vi "PrefDialog.vi"(8 "error in (no error)":errorcluster, 11 "MyPluginsBase in":refnum<class "AcPwrBase.lvclass">) -> (0 "error out":errorcluster, 1 "Save As":bool, 2 "Changed":bool, 3 "MyPluginsBase out":refnum<class "AcPwrBase.lvclass">)   [LabVIEW 2018, in "AcPwrPlugins.lvlib" / "AcPwrBase.lvclass"]
uses:
  AcPwrBase.lvclass
  C:/Program Files (x86)/National Instruments/LabVIEW 2018/user.lib/NIST/BaseClasses/BasePlugin_class/BasePlugin.lvclass
  TypeDefs/BaseConfig.ctl
  TypeDefs/Phase.ctl
  TypeDefs/BaseMeasurements.ctl
  TypeDefs/MeasType.ctl
  <userlib>/NIST/BaseClasses/BasePlugin_class/BasePlugin.lvclass/BasePlugin.ctl
  AcPwrBase.lvclass/AcPwrBase.ctl
  FGen/MemberClasses/FunctionBaseClass/FunctionBase.lvclass
  <userlib>/NIST/BaseClasses/BasePlugin_class/Accessors/Read PluginIniFilePath.vi
  Accessors/Read BaseConfig.vi
  Accessors/Read FunctionINIFilePath.vi
  Accessors/Read RefreshTime.vi
  Accessors/Read BaseMeasurements.vi
  Accessors/Read FunctionClass.vi
  Accessors/Write FunctionClass.vi
  Accessors/Write FunctionINIFilePath.vi
  Accessors/Write BaseConfig.vi
  Accessors/Write RefreshTime.vi
  Accessors/Write BaseMeasurements.vi
  <userlib>/NIST/BaseClasses/BasePlugin_class/Accessors/Write PluginIniFilePath.vi
  <vilib>/Utility/error.llb/Error Cluster From Error Code.vi
  <vilib>/ErrorRing/Error Ring.xnode
  <vilib>/Utility/config.llb/NI_LVConfig.lvlib
  <userlib>/NIST/BaseClasses/Object_class/BaseObject.lvclass
panel:
  in  "BaseMeasurements":T1
  in  "btnSaveAs":bool
  in  "btnSave":bool
  in  "RefreshTime":dbl
  in  "FunctionIniFilePath":path
  in  "btnFuncConfig":bool
  in  "btnCancel":bool
  in  "BaseConfig":T3
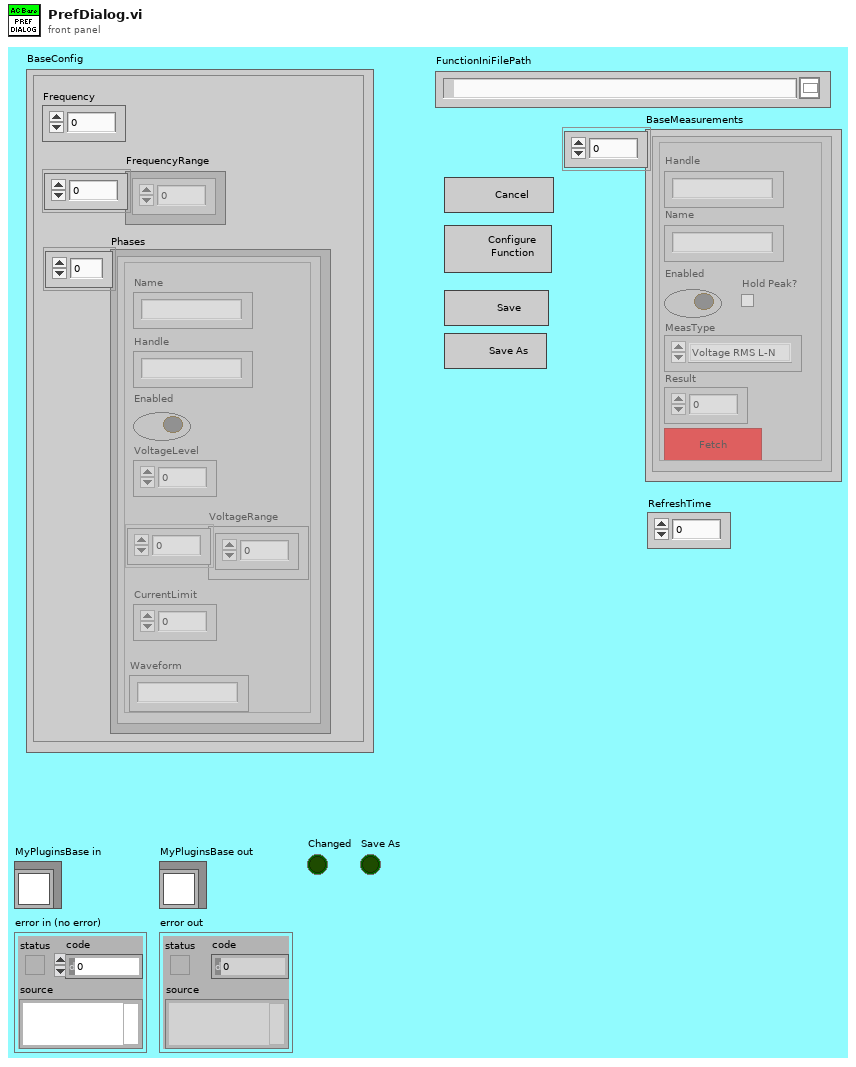
[diagram p1: front panel]
types:
  T1 = typedef "AcPwrPlugins.lvlib/AcPwrBase.lvclass/BaseMeasurements.ctl" = cluster{"Handle":string, "Name":string, "Enabled":bool, "Result":dbl, "MeasType":T2, "btnMeasFetch":bool, "Hold Peak?":bool}[]
  T2 = typedef "AcPwrPlugins.lvlib/AcPwrBase.lvclass/MeasType.ctl" = enum16{"Voltage RMS L-N", "Current RMS", "Frequency", "Voltage DC", "Current DC", "Power Factor", "Current Peak", "Power VA", "Real Power", "Voltage THD", "Voltage EHD", "Voltage OHD", "Current THD", "Current EHD", "Current OHD", "Voltage RMS L-L", "Phase Angle", "Power DC", "Crest Factor"}
  T3 = typedef "AcPwrPlugins.lvlib/AcPwrBase.lvclass/BaseConfig.ctl" = cluster{"Frequency":dbl, "FrequencyRange":dbl[], "Phases":T4[]}
  T4 = typedef "AcPwrPlugins.lvlib/AcPwrBase.lvclass/Phase.ctl" = cluster{"Name":string, "Enabled":bool, "VoltageLevel":dbl, "Handle":string, "VoltageRange":dbl[], "Connected":bool, "CurrentLimit":dbl, "Waveform":string}
  T5 = enum8{"Enabled", "Disabled", "Disabled and Grayed Out"}
  T6 = enum32{"Invalid", "Standard", "Closed", "Hidden", "Minimized", "Maximized"}
  T7 = enum32{"Invalid", "Default", "Floating", "Floating/Auto-Hide", "Modal"}
  T8 = typedef "NI_LVConfig.lvlib/Config Data RefNum.ctl" = refnum<k1>
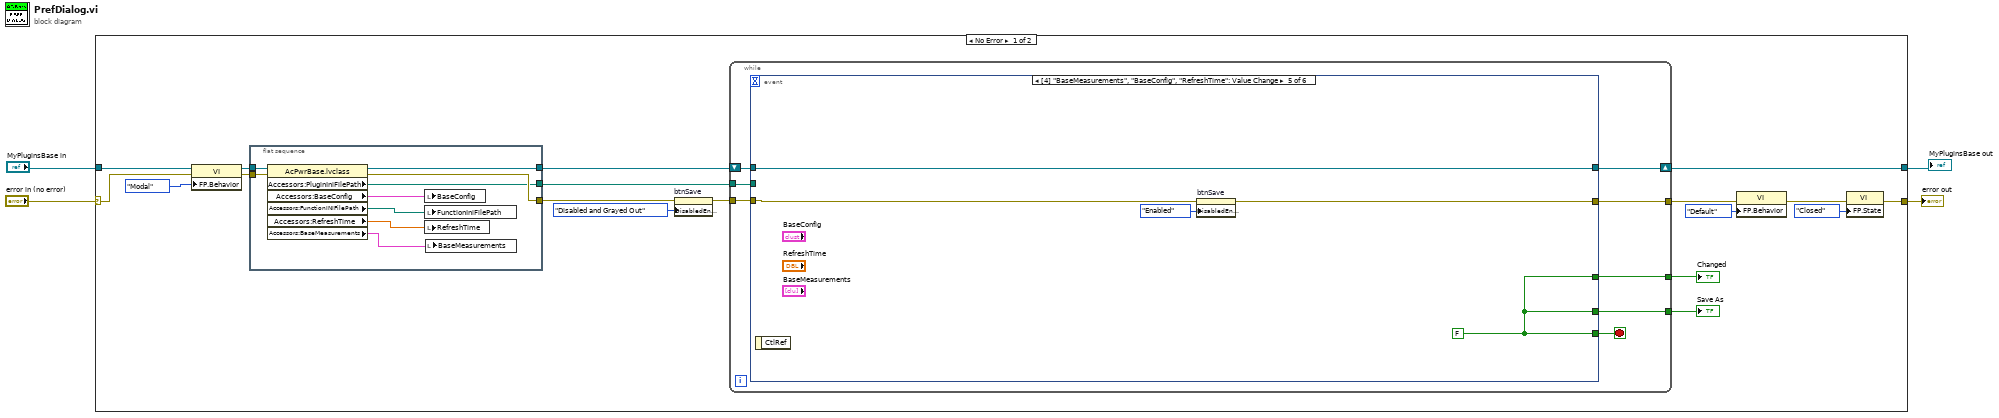
[diagram p0: block diagram]
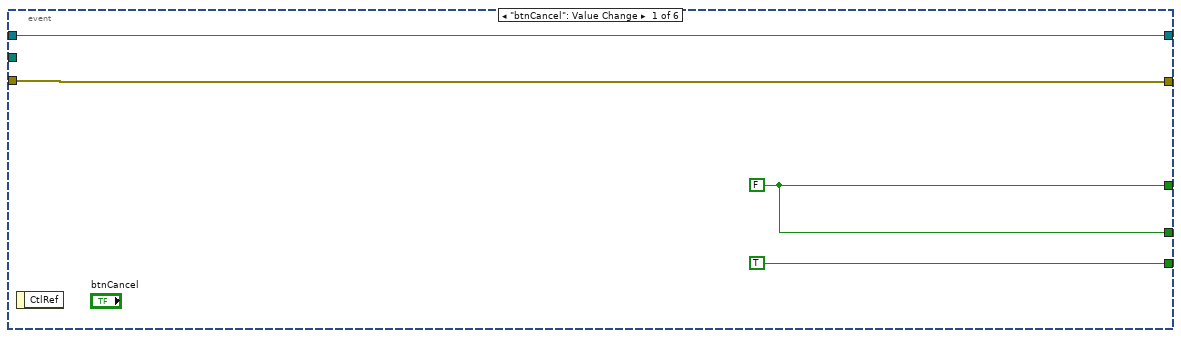
[diagram p2: hidden frame]
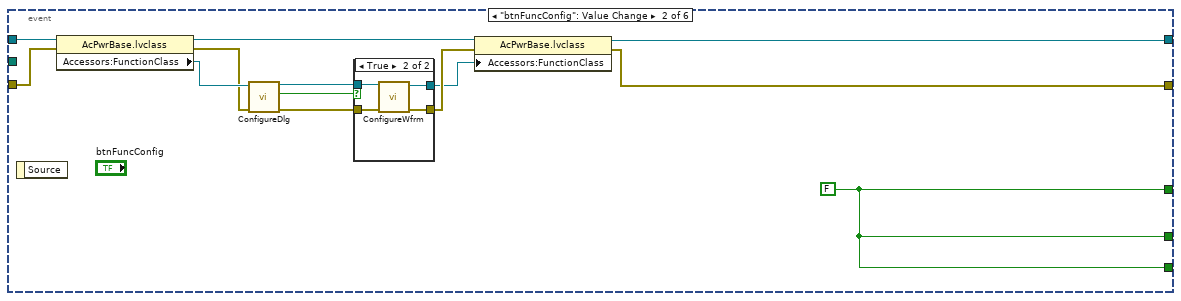
[diagram p3: hidden frame]
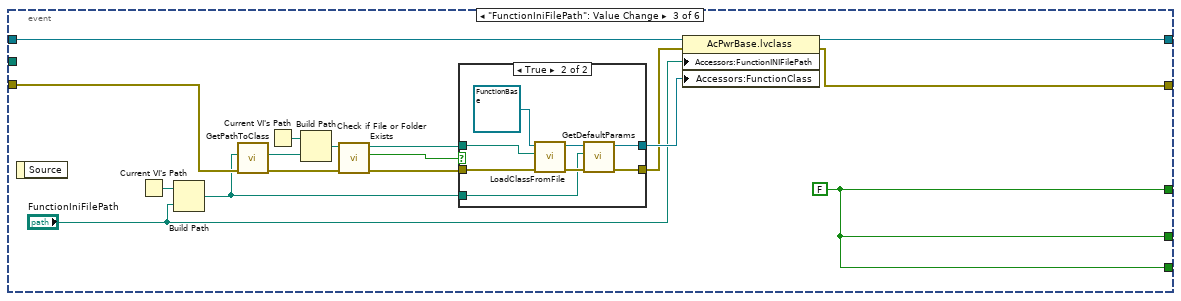
[diagram p5: hidden frame]
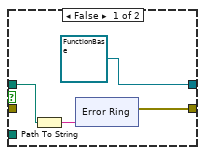
[diagram p6: hidden frame]
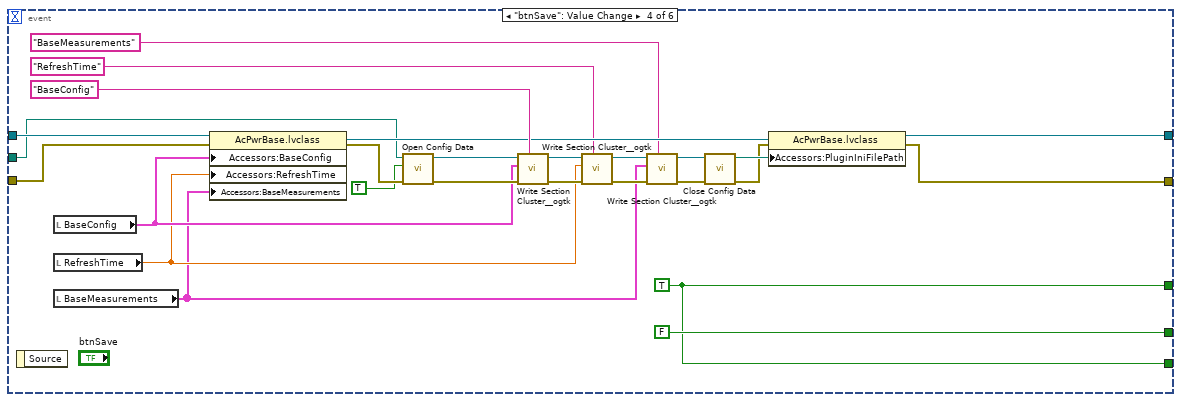
[diagram p7: hidden frame]
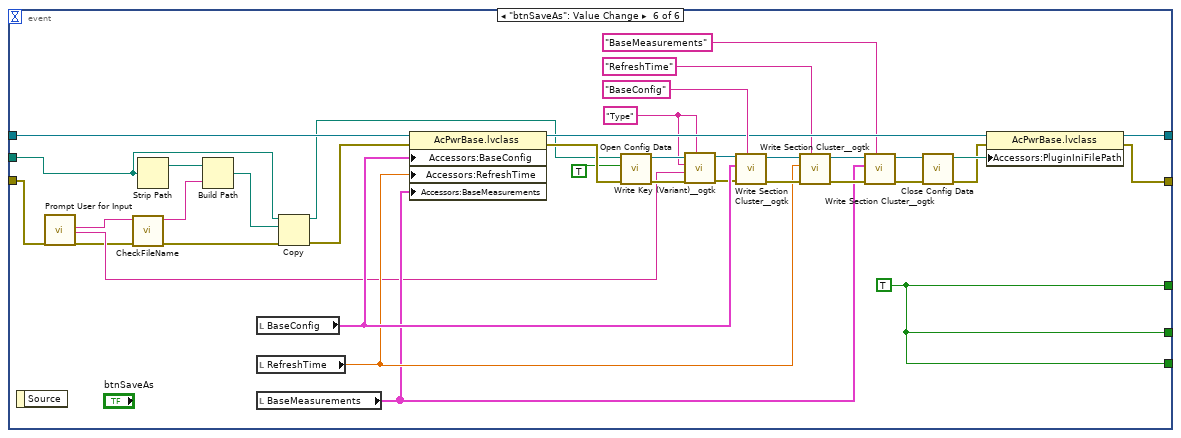
[diagram p8: hidden frame]
diagram:
  n1 = case shown="No Error" "error in (no error)" {
    selector: "error in (no error)" -> [w19 w167]
    tunnel: "MyPluginsBase in" -> [w21 w166]
    tunnel: [w15 w167] -> w2
    tunnel: [w11 w166] -> w1
    frame No Error {
      n2 = property class="VI"(error in=w19, "FP.Behavior"=T7."Modal" ("Front Panel Window:Behavior")) -> (error out=w8:errorcluster)  [unwired: 1 in, 1 out]
      n3 = flat-sequence {
        tunnel: w21 -> [w30]
        tunnel: [w29] -> w20
        tunnel: [w27] -> w7
        tunnel: w8 -> [w28]
        tunnel: [w24] -> w9
        frame #0 {
          n4 = property class="AcPwrBase.lvclass"(reference=w30, error in=w28) -> (reference out=w29:refnum<class "AcPwrBase.lvclass">, error out=w27:errorcluster, "Accessors:PluginIniFilePath"=w24:path, "Accessors:BaseConfig"=w22:T3, "Accessors:FunctionINIFilePath"=w26:path, "Accessors:RefreshTime"=w25:dbl, "Accessors:BaseMeasurements"=w23:T1)
          n5 = local write "BaseConfig"(w22) -> ()
          n6 = local write "FunctionIniFilePath"(w26) -> ()
          n7 = local write "RefreshTime"(w25) -> ()
          n8 = local write "BaseMeasurements"(w23) -> ()
        }
      }
      n9 = property on="btnSave" class="Bool"(error in=w7, "DisabledEnum"=T5."Disabled and Grayed Out" ("Disabled")) -> (error out=w6:errorcluster)  [unwired: 1 in, 1 out]
      n10 = while {
        shift-right: [w37] -> w11
        shift-left: w20 -> [w38]
        tunnel: [w36] -> w17
        tunnel: w6 -> [w35]
        tunnel: [w33] -> w12
        tunnel: [w32] -> w10
        tunnel: w9 -> [w31]
        stop <- w34 stop-if-true
        n11 = event shown="[4] \"BaseMeasurements\", \"BaseConfig\", \"RefreshTime\": Value Change" {
          selector: _ -> [_ _ _ _ _ _]
          dyn-events: _ -> [_ _ _ _ _ _]
          timeout: _ -> [_ _ _ _ _ _]
          tunnel: w38 -> [w42 w55 w77 w106 w127 w151]
          tunnel: [w42 w54 w76 w117 w127 w161] -> w37
          tunnel: [w41 w49 w78 w104 w125 w149] -> w36
          tunnel: w35 -> [w41 w52 w75 w107 w126 w142]
          tunnel: [TRUE w43 w62 w101 w128 w129] -> w34
          tunnel: [w39 w43 w62 w101 w128 w129] -> w33
          tunnel: [w39 w43 w62 FALSE w128 w129] -> w32
          tunnel: w31 -> [_ _ _ w102 _ w141]
          event "btnCancel": Value Change {
            w39 = FALSE
            n12 = event-data() -> ()  [unwired: 1 in, 1 out]
          }
          event "btnFuncConfig": Value Change {
            w43 = FALSE
            n13 = event-data() -> ()  [unwired: 1 in, 1 out]
            n14 = property class="AcPwrBase.lvclass"(reference=w55, error in=w52) -> (reference out=w53:refnum<class "AcPwrBase.lvclass">, error out=w45:errorcluster, "Accessors:FunctionClass"=w46:refnum<class "FunctionBase.lvclass">)
            n15 = call-dynamic "ConfigureDlg.vi"("error in (no error)"=w45, "FunctionBase in"=w46) -> ("error out"=w44:errorcluster, "Changed"=w48:bool, "FunctionBase out"=w47:refnum<class "FunctionBase.lvclass">)  [unwired: 7 in]
            n16 = case shown="True" w48 {
              tunnel: w44 -> [w56 w58]
              tunnel: w47 -> [w57 w61]
              tunnel: [w56 w60] -> w51
              tunnel: [w57 w59] -> w50
              frame False {
              }
              frame True {
                n17 = call-dynamic "ConfigureWfrm.vi"("error in (no error)"=w58, "FunctionBase in"=w61) -> ("error out"=w60:errorcluster, "FunctionBase out"=w59:refnum<class "FunctionBase.lvclass">)  [unwired: 8 in]
              }
            }
            n18 = property class="AcPwrBase.lvclass"(reference=w53, error in=w51, "Accessors:FunctionClass"=w50) -> (reference out=w54:refnum<class "AcPwrBase.lvclass">, error out=w49:errorcluster)
          }
          event "FunctionIniFilePath": Value Change {
            w62 = FALSE
            n19 = event-data() -> ()  [unwired: 1 in, 1 out]
            n20 = Current VI's Path() -> (path=w65:path)
            n21 = Build Path(base path=w65, name or relative path="FunctionIniFilePath") -> (appended path=w63:path)
            n22 = call <userlib>:"GetPathToClass.vi"("error in (no error)"=w75, "configuration file path"=w63) -> ("error IO"=w71:errorcluster, "PathToClass"=w73:path)  [unwired: 8 in]
            n23 = Current VI's Path() -> (path=w74:path)
            n24 = Build Path(base path=w74, name or relative path=w73) -> (appended path=w72:path)
            n25 = call <vilib>:"Check if File or Folder Exists.vi"("error in (no error)"=w71, "path"=w72) -> ("error out"=w68:errorcluster, "file or folder exists?"=w67:bool, "dup path"=w66:path)  [unwired: 7 in]
            n26 = case shown="True" w67 {
              tunnel: [w81 w92] -> w69
              tunnel: w68 -> [_ w97]
              tunnel: w66 -> [w80 w96]
              tunnel: [refnum<class "FunctionBase.lvclass"> refnum ("Functions.lvlib:FunctionBase.lvclass") w91] -> w70
              tunnel: w63 -> [_ w90]
              frame False {
                n27 = Path To String(path=w80) -> (string=w82:string)
                n28 = xnode "Error Ring"("parameter 0"=w82) -> ("error out"=w81:errorcluster)
              }
              frame True {
                n29 = call-dynamic "LoadClassFromFile.vi"("error in (no error)"=w97, "class path"=w96, "reference in"=refnum<class "FunctionBase.lvclass"> refnum ("Functions.lvlib:FunctionBase.lvclass")) -> ("error out"=w94:errorcluster, "reference out"=w93:refnum<class "FunctionBase.lvclass">)  [unwired: 7 in]
                n30 = call-dynamic "GetDefaultParams.vi"("error in (no error)"=w94, "Path"=w90, "FunctionBase in"=w93) -> ("error out"=w92:errorcluster, "FunctionBase out"=w91:refnum<class "FunctionBase.lvclass">)  [unwired: 7 in]
              }
            }
            n31 = property class="AcPwrBase.lvclass"(reference=w77, error in=w69, "Accessors:FunctionINIFilePath"="FunctionIniFilePath", "Accessors:FunctionClass"=w70) -> (reference out=w76:refnum<class "AcPwrBase.lvclass">, error out=w78:errorcluster)
          }
          event "btnSave": Value Change {
            w101 = TRUE
            n32 = event-data() -> ()  [unwired: 1 in, 1 out]
            n33 = local read "BaseConfig"() -> (w100:T3)
            n34 = local read "RefreshTime"() -> (w99:dbl)
            n35 = local read "BaseMeasurements"() -> (w98:T1)
            n36 = property class="AcPwrBase.lvclass"(reference=w106, error in=w107, "Accessors:BaseConfig"=w100, "Accessors:RefreshTime"=w99, "Accessors:BaseMeasurements"=w98) -> (reference out=w116:refnum<class "AcPwrBase.lvclass">, error out=w123:errorcluster)
            n37 = call <vilib>:"Open Config Data.vi"("error in (no error)"=w123, "create file if necessary (T)"=TRUE, "configuration file path"=w102) -> ("error out"=w122:errorcluster, "refnum"=w121:T8)  [unwired: 6 in, 1 out]
            n38 = call <userlib>:"Write Section Cluster__ogtk.vi"("section (optional)"="BaseConfig", "error in (no error)"=w122, "Section Formatted Cluster"=w100, "refnum"=w121) -> ("error out"=w115:errorcluster, "dup refnum"=w114:T8)  [unwired: 6 in]
            n39 = call <userlib>:"Write Section Cluster__ogtk.vi"("section (optional)"="RefreshTime", "error in (no error)"=w115, "Section Formatted Cluster"=w99, "refnum"=w114) -> ("error out"=w112:errorcluster, "dup refnum"=w110:T8)  [unwired: 6 in]
            n40 = call <userlib>:"Write Section Cluster__ogtk.vi"("section (optional)"="BaseMeasurements", "error in (no error)"=w112, "Section Formatted Cluster"=w98, "refnum"=w110) -> ("error out"=w111:errorcluster, "dup refnum"=w109:T8)  [unwired: 6 in]
            n41 = call <vilib>:"Close Config Data.vi"("error in (no error)"=w111, "refnum"=w109) -> ("error out"=w105:errorcluster, "file path"=w118:path)  [unwired: 8 in]
            n42 = property class="AcPwrBase.lvclass"(reference=w116, error in=w105, "Accessors:PluginIniFilePath"=w118) -> (reference out=w117:refnum<class "AcPwrBase.lvclass">, error out=w104:errorcluster)
          }
          event "RefreshTime": Value Change {
            w128 = FALSE
            n43 = event-data() -> ()  [unwired: 1 in, 1 out]
            n44 = property on="btnSave" class="Bool"(error in=w126, "DisabledEnum"=T5."Enabled" ("Disabled")) -> (error out=w125:errorcluster)  [unwired: 1 in, 1 out]
          }
          event "btnSaveAs": Value Change {
            w134 = "Type" ("section (optional)")
            w129 = TRUE
            n45 = event-data() -> ()  [unwired: 1 in, 1 out]
            n46 = call "Prompt User for Input"("error in (no error)"=w142) -> ("File Name"=w133:string, "PluginType"=w135:string, "error out"=w132:errorcluster)  [unwired: 15 in, 1 out]
            n47 = call "CheckFileName.vi"("Error In"=w132, "File Name in"=w133) -> ("Error Out"=w130:errorcluster, "File Name out"=w131:string)  [unwired: 8 in]
            n48 = Strip Path(path=w141) -> (stripped path=w145:path)  [unwired: 1 out]
            n49 = Build Path(base path=w145, name or relative path=w131) -> (appended path=w144:path)
            n50 = local read "BaseConfig"() -> (w148:T3)
            n51 = local read "RefreshTime"() -> (w147:dbl)
            n52 = local read "BaseMeasurements"() -> (w146:T1)
            n53 = Copy(8:w130, 10:w144, 11:w141) -> (0:w143:errorcluster, 3:w140:path)  [unwired: 2 in, 1 out]
            n54 = property class="AcPwrBase.lvclass"(reference=w151, error in=w143, "Accessors:BaseConfig"=w148, "Accessors:RefreshTime"=w147, "Accessors:BaseMeasurements"=w146) -> (reference out=w160:refnum<class "AcPwrBase.lvclass">, error out=w165:errorcluster)
            n55 = call <vilib>:"Open Config Data.vi"("error in (no error)"=w165, "create file if necessary (T)"=TRUE, "configuration file path"=w140) -> ("error out"=w137:errorcluster, "refnum"=w136:T8)  [unwired: 6 in, 1 out]
            n56 = call <userlib>:"Write Key (Variant)__ogtk.vi"("section"=w134, "error in (no error)"=w137, "key-value"=w135, "key (optional)"=w134, "refnum"=w136) -> ("error out"=w139:errorcluster, "refnum out"=w138:T8)  [unwired: 5 in]
            n57 = call <userlib>:"Write Section Cluster__ogtk.vi"("section (optional)"="BaseConfig", "error in (no error)"=w139, "Section Formatted Cluster"=w148, "refnum"=w138) -> ("error out"=w159:errorcluster, "dup refnum"=w158:T8)  [unwired: 6 in]
            n58 = call <userlib>:"Write Section Cluster__ogtk.vi"("section (optional)"="RefreshTime", "error in (no error)"=w159, "Section Formatted Cluster"=w147, "refnum"=w158) -> ("error out"=w156:errorcluster, "dup refnum"=w154:T8)  [unwired: 6 in]
            n59 = call <userlib>:"Write Section Cluster__ogtk.vi"("section (optional)"="BaseMeasurements", "error in (no error)"=w156, "Section Formatted Cluster"=w146, "refnum"=w154) -> ("error out"=w155:errorcluster, "dup refnum"=w153:T8)  [unwired: 6 in]
            n60 = call <vilib>:"Close Config Data.vi"("error in (no error)"=w155, "refnum"=w153) -> ("error out"=w150:errorcluster, "file path"=w162:path)  [unwired: 8 in]
            n61 = property class="AcPwrBase.lvclass"(reference=w160, error in=w150, "Accessors:PluginIniFilePath"=w162) -> (reference out=w161:refnum<class "AcPwrBase.lvclass">, error out=w149:errorcluster)
          }
        }
      }
      "Changed" <- w12
      "Save As" <- w10
      n62 = property class="VI"(error in=w17, "FP.Behavior"=T7."Default" ("Front Panel Window:Behavior")) -> (error out=w16:errorcluster)  [unwired: 1 in, 1 out]
      n63 = property class="VI"(error in=w16, "FP.State"=T6."Closed" ("Front Panel Window:State")) -> (error out=w15:errorcluster)  [unwired: 1 in, 1 out]
    }
    frame Error {
    }
  }
  "error out" <- w2
  "MyPluginsBase out" <- w1
